vi "Matrix_host.vi"() -> ()   [LabVIEW 2013]
uses:
  <vilib>/userdefined/High Color/nirio_resource_hc.ctl
  <vilib>/FPGAPlugInAG/PXI-7953R/niLvFpga_Open_PXI-7953R.vi
  <vilib>/rvi/interface/common/dynamic/niFpgaDynamicAddResources.vi
  <vilib>/FPGAPlugInAG/Dynamic/niLvFpga_Reset_Dynamic.vi
  <vilib>/FPGAPlugInAG/Dynamic/niLvFpga_Run_Dynamic.vi
  <vilib>/rvi/interface/common/niFpgaWaitOnOcc.vi
  <vilib>/Utility/error.llb/Error Cluster From Error Code.vi
  <vilib>/rvi/errors/niLvFpgaAdjustHostInterfaceError.vi
  <vilib>/FPGAPlugInAG/Dynamic/niLvFpga_Close_Dynamic.vi
  <vilib>/rvi/interface/nirviOpenFPGA/nirviOpenFPGA.xnode
  FPGA Bitfiles/Matrix_Writetarget_Matrixtarget_Bx2+jPDz+iI.lvbitx
  <vilib>/rvi/interface/nirviMethod/nirviMethod.xnode
  <vilib>/rvi/interface/nirviReadWriteControl/nirviReadWriteControl.xnode
  <vilib>/rvi/interface/nirviCloseFPGA/nirviCloseFPGA.xnode
  NiFpgaLv.dll
  <vilib>/rvi/interface/Simulation/niFpgaSimulationCallBeginRW.vi
panel:
  in  "1_EXTCLK_divider":i16=4
  out "ACK":u8 format="%8b"
  out "ACK":bool[](array[boolean])
  in  "100_Sclk_divider":i32=100
  in  "75_Stop":i16=75
  in  "10_Rise/Fall divider":i32=10
  in  "0_WE divider":i32
  in  "53":i16=53
  in  "35":i16=35
  in  "17":i16=17
  in  "71":i16=71
  in  "72":i16=72
  in  "18":i16=18
  in  "36":i16=36
  in  "54":i16=54
  out "ArrayUp":u64
  out "ArrayLow":u64
  in  "DataLow":u8=18 format="%x"
  in  "Device":u8=186 format="%x"
  in  "DataUp":u8=54 format="%x"
  in  "Reg":u8=9 format="%x"
  in  "Send":bool=TRUE
  in  "ПЛИС":T1="PXI1Slot5"
  in  "Стоп":bool
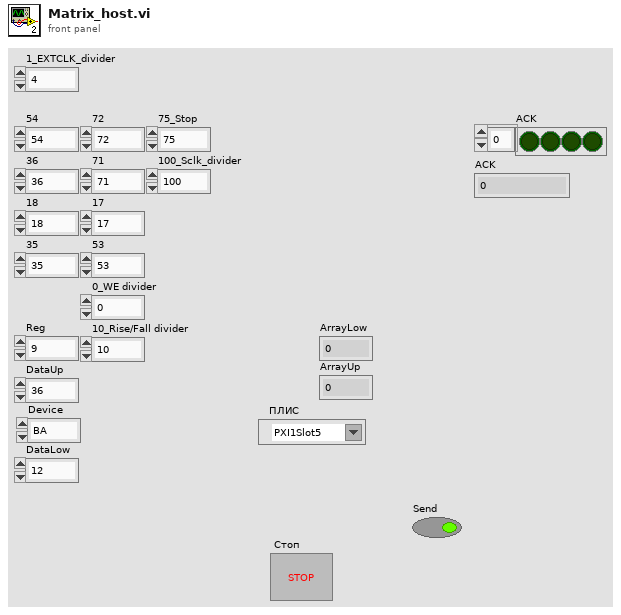
[diagram p1: front panel]
types:
  T1 = typedef "nirio_resource_hc.ctl" = tag
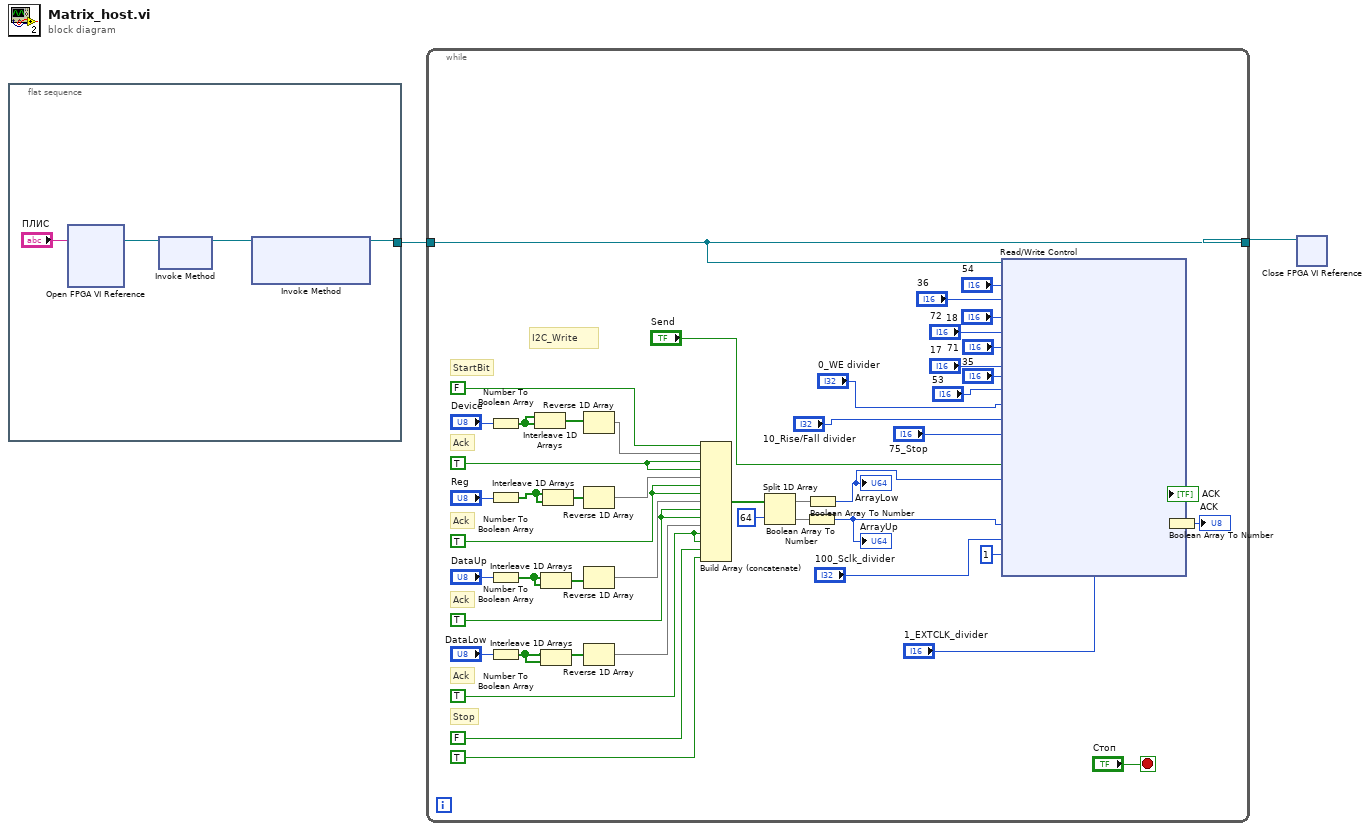
[diagram p0: block diagram]
diagram:
  n1 = flat-sequence {
    tunnel: [w6] -> w2
    frame #0 {
      n2 = xnode "Open FPGA VI Reference"("resource name"="ПЛИС") -> ("FPGA VI Reference Out"=w4:refnum<k20>)  [unwired: 1 in, 1 out]
      n3 = xnode "Invoke Method"("FPGA VI Reference In"=w4) -> ("FPGA VI Reference Out"=w3:refnum<k20>)  [unwired: 1 in, 1 out]
      n4 = xnode "Invoke Method"("FPGA VI Reference In"=w3) -> ("FPGA VI Reference Out"=w6:refnum<k20>)  [unwired: 2 in, 1 out]
    }
  }
  n5 = while {
    tunnel: w2 -> [w53]
    tunnel: [w53] -> w1
    stop <- "Стоп" stop-if-true
    w40 = TRUE
    w43 = TRUE
    w46 = TRUE
    w49 = TRUE
    # "Stop"
    # "Ack"
    # "Ack"
    # "Ack"
    # "Ack"
    # "StartBit"
    # "I2C_Write"
    n6 = Number To Boolean Array(number="Device") -> (Boolean array=w37:bool[])
    n7 = Number To Boolean Array(number="Reg") -> (Boolean array=w31:bool[])
    n8 = Number To Boolean Array(number="DataUp") -> (Boolean array=w32:bool[])
    n9 = Number To Boolean Array(number="DataLow") -> (Boolean array=w30:bool[])
    n10 = Interleave 1D Arrays(w37, w37) -> (w36:bool[])
    n11 = Interleave 1D Arrays(w32, w32) -> (w33:bool[])
    n12 = Interleave 1D Arrays(w30, w30) -> (w35:bool[])
    n13 = Interleave 1D Arrays(w31, w31) -> (w34:bool[])
    n14 = Reverse 1D Array(array=w36) -> (reversed array=w51:bool[])
    n15 = Reverse 1D Array(array=w34) -> (reversed array=w48:bool[])
    n16 = Reverse 1D Array(array=w33) -> (reversed array=w44:bool[])
    n17 = Reverse 1D Array(array=w35) -> (reversed array=w42:bool[])
    n18 = Build Array (concatenate)(FALSE, w51, w49, w49, w48, w46, w46, w44, w43, w43, w42, w40, w40, FALSE, TRUE) -> (w28:bool[])
    n19 = Split 1D Array(array=w28, index=u64 64) -> (first subarray=w27:bool[], second subarray=w26:bool[])
    n20 = Boolean Array To Number(Boolean array=w26) -> (number=w12:u64)
    "ArrayUp" <- w12
    n21 = Boolean Array To Number(Boolean array=w27) -> (number=w13:u64)
    "ArrayLow" <- w13
    n22 = xnode "Read/Write Control"("FPGA VI Reference In"=w53, "54"="54", "36"="36", "18"="18", "72"="72", "71"="71", "17"="17", "35"="35", "53"="53", "0_WE divider"="0_WE divider", "10_Rise/Fall divider"="10_Rise/Fall divider", "75_Stop"="75_Stop", "Send_Request"="Send", "DataLow"=w13, "DataUp"=w12, "100_Sclk_divider"="100_Sclk_divider", "IO Module\\Local_Supply_Select"=u8 1 ("IO Module\\Local_Supply_Select"), "1_EXTCLK_divider"="1_EXTCLK_divider") -> ("ACK"=w10:bool[])  [unwired: 1 in, 4 out]
    "ACK" <- w10
    n23 = Boolean Array To Number(Boolean array=w10) -> (number=→"ACK":u8)
  }
  n24 = xnode "Close FPGA VI Reference"("FPGA VI Reference In"=w1) -> ()  [unwired: 1 in, 1 out]
